vi "Helper commandType.vi"(8 "error in (no error)":errorcluster, 11 "CommandType":i32(ring)=-1 items=["Text"=1, "StoredProcedure"=4, "TableDirect"=512]) -> (0 "error out":errorcluster, 3 ".NET Refnum out":refnum<k24>)   [LabVIEW 2020, in "ORM_Dapper.lvlib" / "DapperMapper.lvclass"]
uses:
  DapperMapper.lvclass
  System.Data
  DapperMapper.lvclass/DapperMapper.ctl
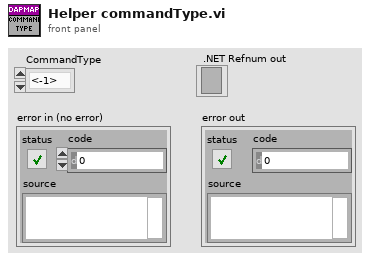
[diagram p1: front panel]
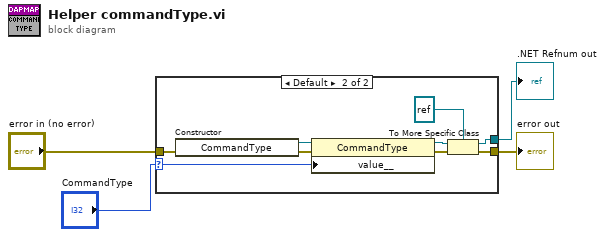
[diagram p0: block diagram]
diagram:
  n1 = case shown="Default" "CommandType" {
    selector: "CommandType" -> [_ w14]
    tunnel: [_ w12] -> w2
    tunnel: "error in (no error)" -> [w5 w7]
    tunnel: [w5 w6] -> w4
    frame -1 {
    }
    frame Default {
      n2 = constructor class="CommandType"(error in=w7) -> (reference out=w9:refnum<k24>, error out=w8:errorcluster)  [unwired: 2 in, 1 out]
      n3 = property class="CommandType"(reference=w9, error in=w8, "value__"=w14) -> (reference out=w13:refnum<k24>, error out=w10:errorcluster)
      n4 = To More Specific Class(target class=refnum<k24> refnum ("commandType"), reference=w13, error in=w10) -> (specific class reference=w12:refnum<k24>, error out=w6:errorcluster)
    }
  }
  "error out" <- w4
  ".NET Refnum out" <- w2
